vi "I_M_Card_Read.vi"(8 "error in (no error)":errorcluster, 10 "Card Read":bool, 11 "Interface_Display_Console in":refnum<class "Interface_Display_Console.lvclass">) -> (0 "error out":errorcluster, 3 "Interface_Display_Console out":refnum<class "Interface_Display_Console.lvclass">)   [LabVIEW 2025, in "Display_Console.lvlib" / "Interface_Display_Console.lvclass"]
uses:
  Interface_Display_Console.lvclass
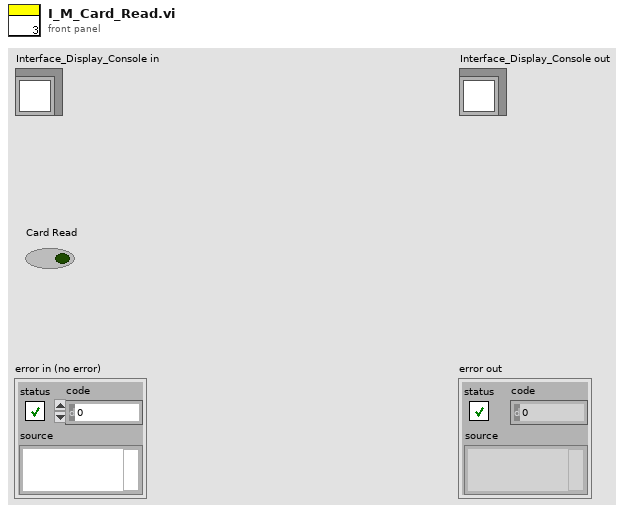
[diagram p1: front panel]
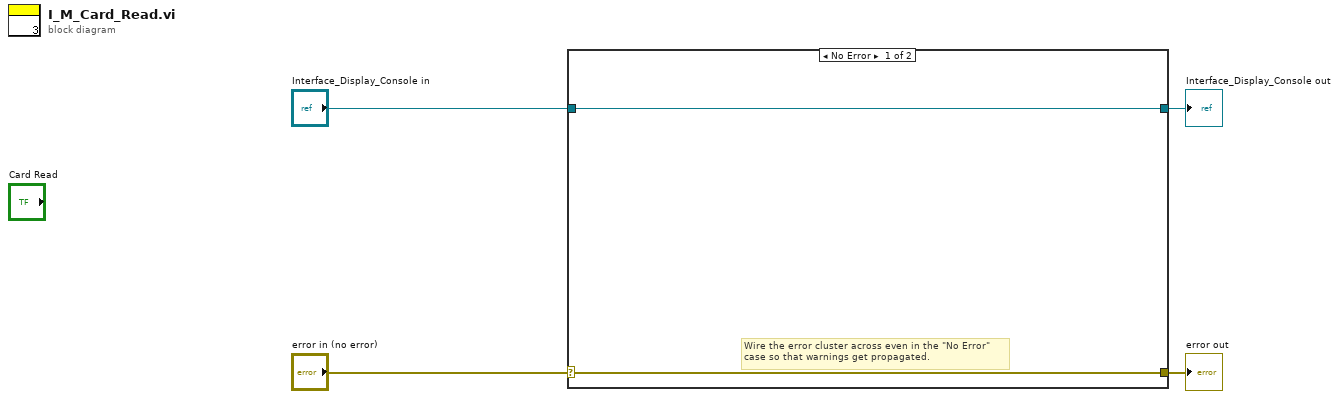
[diagram p0: block diagram]
diagram:
  n1 = case shown="No Error" "error in (no error)" {
    selector: "error in (no error)" -> [w5 w8]
    tunnel: [w5 w8] -> w3
    tunnel: [w6 w7] -> w1
    tunnel: "Interface_Display_Console in" -> [w6 w7]
    frame No Error {
      # "Wire the error cluster across even in the \"No Error\"\ncase so that warnings get propagated."
    }
    frame Error {
    }
  }
  "error out" <- w3
  "Interface_Display_Console out" <- w1
